vi "Trainning body.vi"(8 "error in":errorcluster, 11 "BioInfo":T1) -> (0 "error out":errorcluster, 3 "BioInfo out":T1={"Heart Rate"=90, "Age"=25, "Sex"=enum."Male", "Level"=0})   [LabVIEW 2016]
uses:
  Control/Bio_Information.ctl
panel:
  in  "Level":u8
  in  "Cancel Button":bool
  in  "OK Button":bool
  out "Boolean":bool=TRUE caption="Bio- Information"
  in  "Sex":enum16{"Male", "Female"}(ring)
  in  "Age":u8
  in  "Heart Rate Threshold":u8
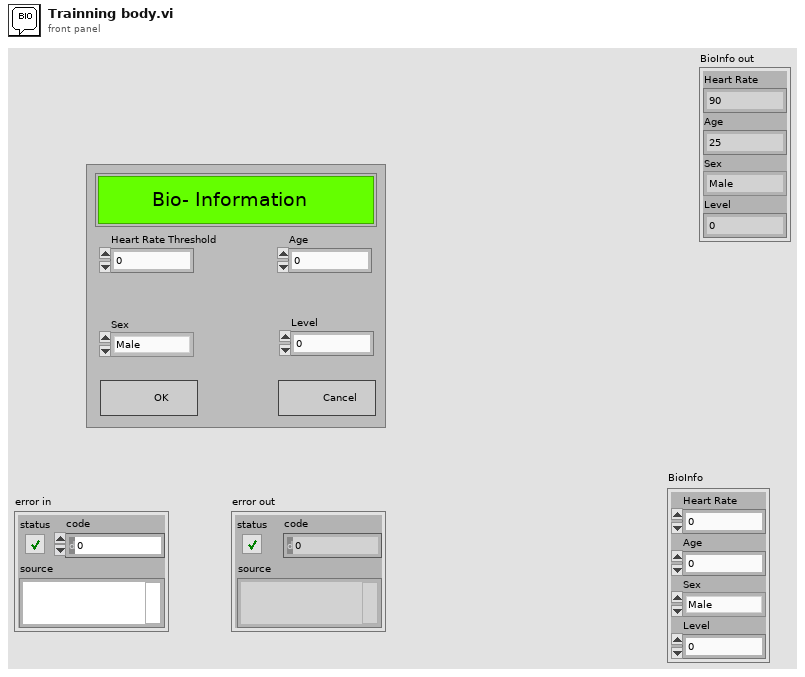
[diagram p1: front panel]
types:
  T1 = typedef "Bio_Information.ctl" = cluster{"Heart Rate":u8, "Age":u8, "Sex":enum16{"Male", "Female"}, "Level":u8}
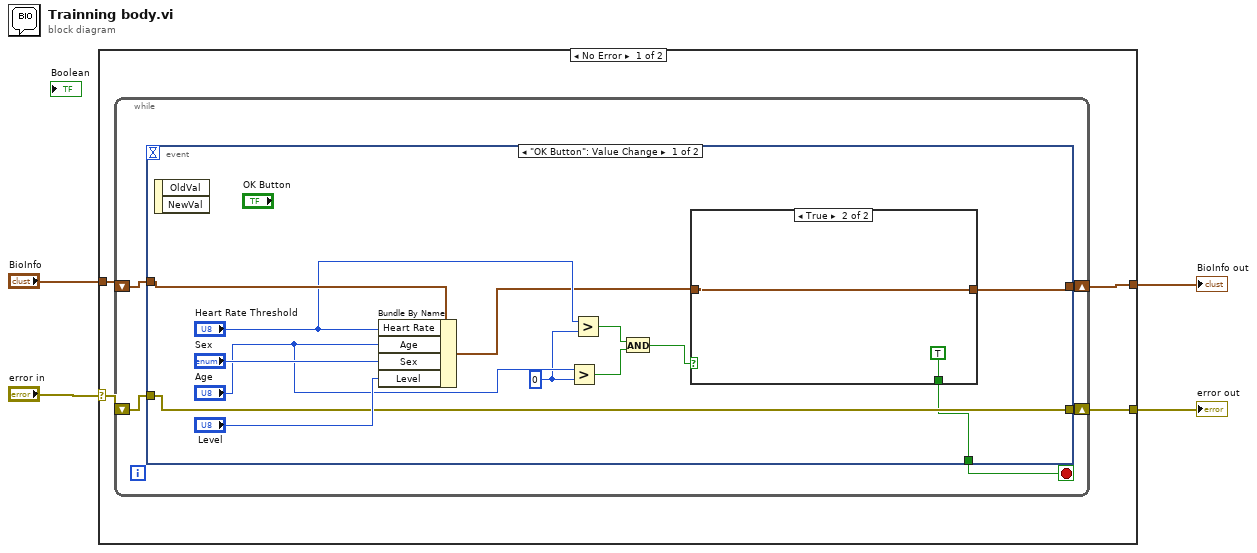
[diagram p0: block diagram]
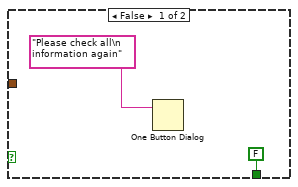
[diagram p2: hidden frame]
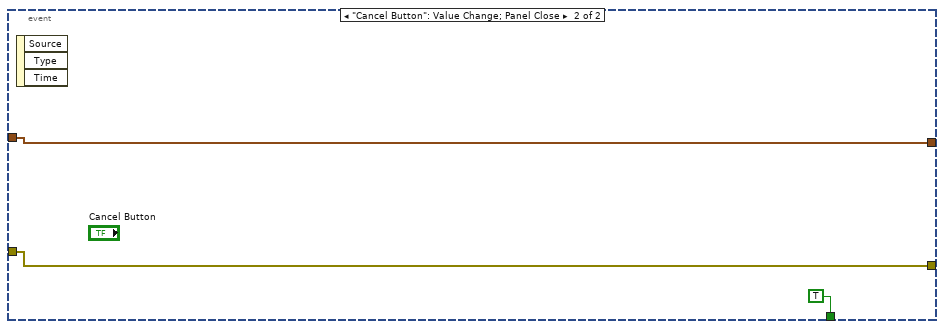
[diagram p3: hidden frame]
diagram:
  n1 = case shown="No Error" "error in" {
    selector: "error in" -> [w6 w35]
    tunnel: [w5 w35] -> w3
    tunnel: [w8 w34] -> w1
    tunnel: "BioInfo" -> [w7 w34]
    frame No Error {
      n2 = while {
        shift-right: [w13] -> w8
        shift-left: w7 -> [w12]
        shift-right: [w10] -> w5
        shift-left: w6 -> [w11]
        stop <- w9 stop-if-true
        n3 = event shown="[0] \"OK Button\": Value Change" {
          selector: _ -> [_ _]
          dyn-events: _ -> [_ _]
          timeout: _ -> [_ _]
          tunnel: [w16 w33] -> w13
          tunnel: w12 -> [w24 w33]
          tunnel: w11 -> [w23 w32]
          tunnel: [w23 w32] -> w10
          tunnel: [w14 TRUE] -> w9
          event "OK Button": Value Change {
            w18 = u8 0 ("y")
            n4 = event-data() -> ()  [unwired: 1 in, 2 out]
            n5 = Bundle By Name(cluster=w24, "Heart Rate"="Heart Rate Threshold", "Age"="Age", "Sex"="Sex", "Level"="Level") -> (w17:T1)
            n6 = Greater?(x="Age", y=w18) -> (0:w21:bool)
            n7 = Greater?(x="Heart Rate Threshold", y=w18) -> (0:w22:bool)
            n8 = And(x=w22, y=w21) -> (x .and. y?=w15:bool)
            n9 = case shown="True" w15 {
              tunnel: w17 -> [_ w30]
              tunnel: [_ w30] -> w16
              tunnel: [FALSE TRUE] -> w14
              frame False {
                n10 = One Button Dialog(message="Please check all\n information again") -> ()  [unwired: 1 in, 1 out]
              }
              frame True {
              }
            }
          }
          event "Cancel Button": Value Change; Panel Close {
            n11 = event-data() -> ()  [unwired: 1 in, 3 out]
          }
        }
      }
    }
    frame Error {
    }
  }
  "error out" <- w3
  "BioInfo out" <- w1
